vi "SLSC Separate Channel Configuration.vi"(0 "Encoded String":string) -> (3 "Default Array Data":dbl[](array[numeric]), 4 "Channel":string, 6 "output cluster":T1, 8 "Default Data":dbl, 10 "Type of channel":string, 14 "Unit":string)   [LabVIEW 2015, in "SLSC-12201 DIO System Explorer.lvlib"]
uses:
  <vilib>/NI Veristand/Custom Device API/Custom Device Channel.ctl
  <vilib>/NI Veristand/Custom Device API/Custom Device Channel Type.ctl
  SLSC-12201 DIO System Explorer.lvlib
  <vilib>/NI VeriStand/Custom Device API/Custom Device API.lvlib
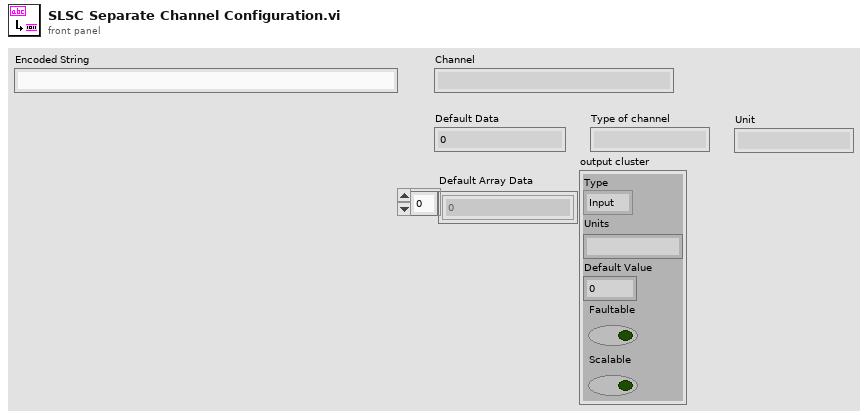
[diagram p1: front panel]
types:
  T1 = typedef "Custom Device API.lvlib/Custom Device Channel.ctl" = cluster{"Type":T2, "Units":string, "Default Value":dbl, "Faultable":bool, "Scalable":bool}
  T2 = typedef "Custom Device API.lvlib/Custom Device Channel Type.ctl" = enum16{"Input", "Output"}
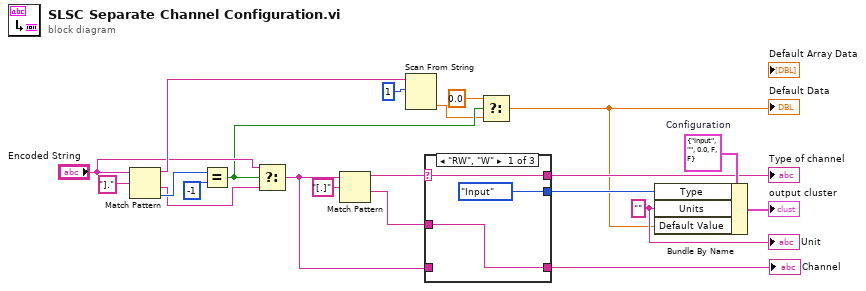
[diagram p0: block diagram]
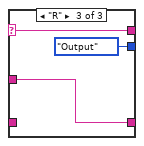
[diagram p3: hidden frame]
diagram:
  w15 = "" ("Units")
  w17 = T1 {"Type"=enum."Input", "Units"="", "Default Value"=0.0, "Faultable"=FALSE, "Scalable"=FALSE}  # Configuration
  n1 = Match Pattern(string="Encoded String", regular expression="].") -> (before substring=w19:string, after substring=w9:string, offset past match=w12:i32)  [unwired: 1 in, 1 out]
  n2 = Equal?(x=w12, y=-1) -> (x = y?=w4:bool)
  n3 = Select(t="Encoded String", s=w4, f=w9) -> (s? t:f=w5:string)
  n4 = Match Pattern(string=w5, regular expression="[.]") -> (before substring=w13:string, after substring=w7:string)  [unwired: 1 in, 2 out]
  n5 = Scan From String(input string=w19, initial scan location=1 ("offset (0)")) -> (output 1=w2:dbl)  [unwired: 3 in, 3 out]
  n6 = case shown="\"RW\", \"W\"" w13 {
    selector: w13 -> [w23 _ w27]
    tunnel: [Custom_Device_Channel_Type."Input" ("Type") _ Custom_Device_Channel_Type."Output" ("Type")] -> w14
    tunnel: [w23 _ w27] -> w8
    tunnel: w7 -> [w22 _ w26]
    tunnel: [w22 w25 w26] -> w6
    tunnel: w5 -> [_ w25 _]
    frame "RW", "W" {
    }
    frame Default {
    }
    frame "R" {
    }
  }
  "Channel" <- w6
  "Type of channel" <- w8
  n7 = Select(t=0.0, s=w4, f=w2) -> (s? t:f=w1:dbl)
  "Default Data" <- w1
  n8 = Bundle By Name(cluster=w17, "Type"=w14, "Units"=w15, "Default Value"=w1) -> (→"output cluster":T1)
  "Unit" <- w15
